vi "Color Get Led Param Fromxy.vi"(0 "smallx":dbl, 5 "smally":dbl, 7 "a_Observer":u8, 11 "error in (no error)":errorcluster) -> (3 "a_CDW out":dbl, 4 "function return":i16, 10 "a_DW out":dbl, 14 "a_Purity out":dbl, 15 "error out":errorcluster)   [LabVIEW 2013, in "AVSirrad.lvlib"]
doc: "DLL_API short int __stdcall Color_GetLedParamFromxy\n(\n double smallx,\n double smally,\n unsigned char a_Observer,\n double *a_DW,\n double *a_CDW,\n double *a_Purity\n);"
uses:
  AVSirrad.lvlib
  AVSIRRAD/Examples/Labview/build/AVSirrad.dll
panel:
  in  "a_Purity":dbl
  in  "a_CDW":dbl
  in  "a_DW":dbl
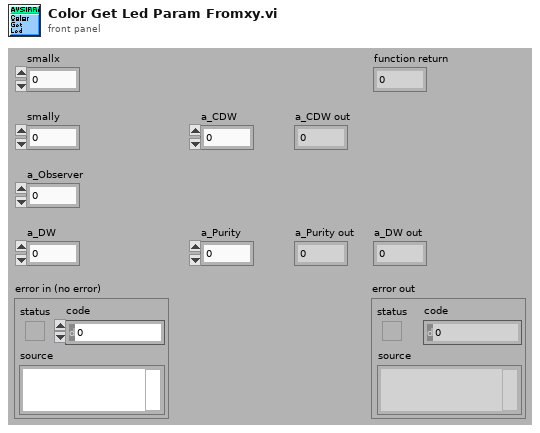
[diagram p1: front panel]
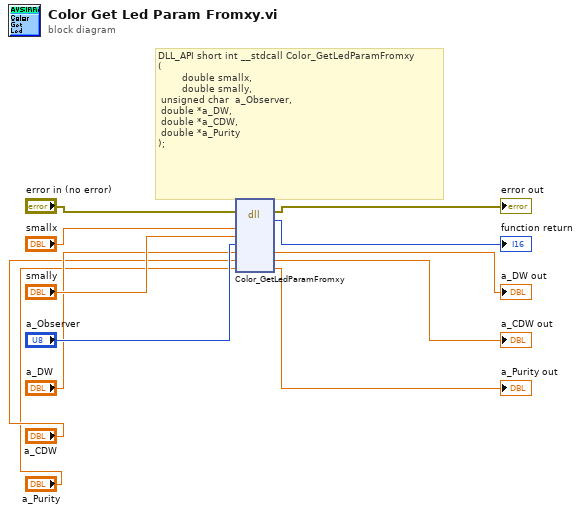
[diagram p0: block diagram]
diagram:
  # "DLL_API short int __stdcall Color_GetLedParamFromxy\n(\n        double smallx,\n        double smally,\n\tunsigned char  a_Observer,\n\tdouble *a_DW,\n\tdouble *a_CDW,\n\tdouble *a_Purity\n);"
  n1 = dll-call lib="C:/AVSIRRAD/Examples/Labview/build/AVSirrad.*" fn="Color_GetLedParamFromxy"(error in="error in (no error)", "smallx"="smallx", "smally"="smally", "a_Observer"="a_Observer", "a_DW"="a_DW", "a_CDW"="a_CDW", "a_Purity"="a_Purity") -> (error out=→"error out":errorcluster, "return type"=→"function return":i16, "a_DW"=→"a_DW out":dbl, "a_CDW"=→"a_CDW out":dbl, "a_Purity"=→"a_Purity out":dbl)  [unwired: 5 in, 1 out]
